vi "Write PWM Outputs.vi"(0 "FPGE Ref":T1, 1 "Frequency":i32, 2 "Controller CMDs IN":dbl[](array[numeric]), 3 "Stagger Counter":i32, 4 "Stagger Time (ms)":i32, 5 "Run Profile":bool) -> (14 "Controller CMDs OUT":dbl[](array[numeric]))   [LabVIEW 2013]
uses:
  Controls/FPGA_Reference.ctl
  <vilib>/Utility/error.llb/Error Cluster From Error Code.vi
  <vilib>/rvi/errors/niLvFpgaAdjustHostInterfaceError.vi
  <vilib>/rvi/interface/nirviReadWriteControl/nirviReadWriteControl.xnode
  FPGA Bitfiles/LSDurabilityMain_Alternate.lvbitx
  NiFpgaLv.dll
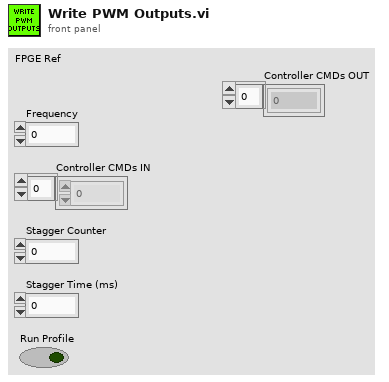
[diagram p1: front panel]
types:
  T1 = typedef "FPGA_Reference.ctl" = refnum<k20>
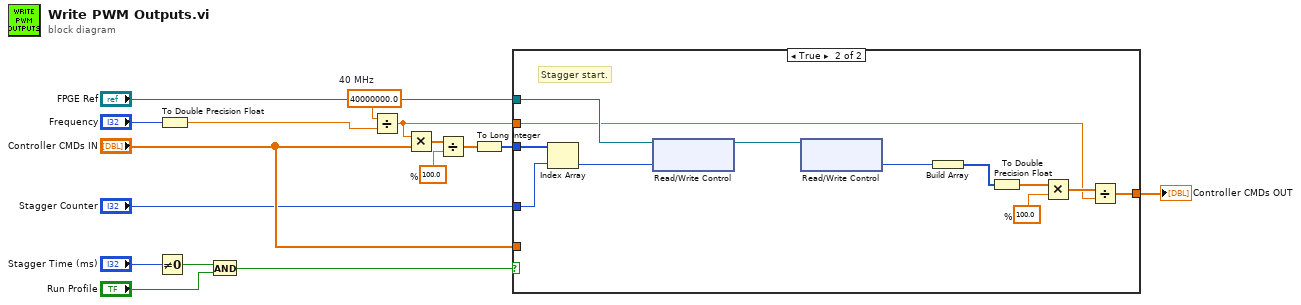
[diagram p0: block diagram]
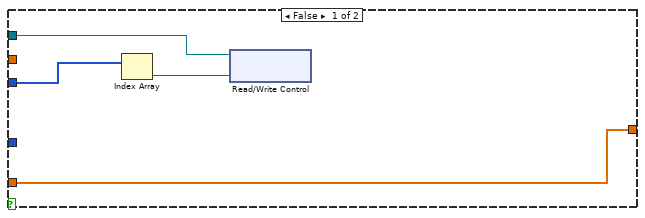
[diagram p2: hidden frame]
diagram:
  w8 = 40000000.0  # 40 MHz
  w10 = 100.0  # %
  n1 = Not Equal To 0?(x="Stagger Time (ms)") -> (x != 0?=w3:bool)
  n2 = To Double Precision Float(number="Frequency") -> (double precision float=w5:dbl)
  n3 = And(x=w3, y="Run Profile") -> (x .and. y?=w1:bool)
  n4 = Divide(x=w8, y=w5) -> (x/y=w14:dbl)
  n5 = Multiply(x=w14, y="Controller CMDs IN") -> (x*y=w11:dbl[])
  n6 = Divide(x=w11, y=w10) -> (x/y=w9:dbl[])
  n7 = To Long Integer(number=w9) -> (32bit integer=w7:i32[])
  n8 = case shown="True" w1 {
    tunnel: w7 -> [w20 w32]
    tunnel: "FPGE Ref" -> [w17 w31]
    tunnel: "Stagger Counter" -> [_ w29]
    tunnel: w14 -> [_ w23]
    tunnel: [w19 w22] -> w15
    tunnel: "Controller CMDs IN" -> [w19 _]
    frame False {
      n9 = Index Array(array=w20) -> (element=w18:i32)  [unwired: 1 in]
      n10 = xnode "Read/Write Control"("FPGA VI Reference In"=w17, "Duty (Ticks)"=w18) -> ()  [unwired: 1 in, 2 out]
    }
    frame True {
      w25 = 100.0  # %
      # "Stagger start."
      n11 = Index Array(array=w32, index=w29) -> (element=w30:i32)
      n12 = xnode "Read/Write Control"("FPGA VI Reference In"=w31, "Duty (Ticks)"=w30) -> ("FPGA VI Reference Out"=w28:T1)  [unwired: 1 in, 1 out]
      n13 = xnode "Read/Write Control"("FPGA VI Reference In"=w28) -> ("Duty (Ticks)"=w21:i32)  [unwired: 1 in, 2 out]
      n14 = Build Array(w21) -> (w27:i32[])
      n15 = To Double Precision Float(number=w27) -> (double precision float=w26:dbl[])
      n16 = Multiply(x=w26, y=w25) -> (x*y=w24:dbl[])
      n17 = Divide(x=w24, y=w23) -> (x/y=w22:dbl[])
    }
  }
  "Controller CMDs OUT" <- w15
